vi "Write Stabilization Data.vi"(8 "error in (no error)":errorcluster, 9 "Output Path":path, 10 "Metadata Array":string[][](array[string]), 11 "Stabilization Data":T1={"Stabilization waveform"={"t0"=timestamp(0 s since 1904-01-01), "dt"=50.0, "Y"=[10.0, 9.0, 8.75, 8.5, 8.25, 8.125, 8.06, 8.03, 8.015, 8.0, 8.0, 8.0]}, "Variation"=0.0, "Stabilized"=FALSE, "Threshold"=0.0, "time to stabilize"=0.0, "3 points"=[], "Sphere Indicator"=enum."Naked Sphere"}) -> (0 "error out":errorcluster)   [LabVIEW 2014, in "Timing and Stabilization.lvlib"]
doc: "Save the details of the stabilization in a *.tdms file"
uses:
  Timing and Stabilization.lvlib
  Stabilization.ctl
  avantesSpectrometer/Acquisition/Sphere Indicator.ctl
  avantesSpectrometer/AvaSpec.lvlib
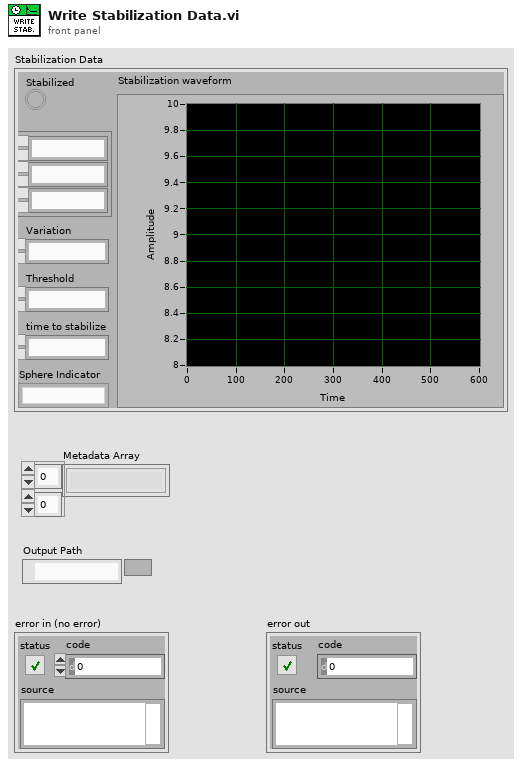
[diagram p1: front panel]
types:
  T1 = typedef "Timing and Stabilization.lvlib/Stabilization.ctl" = cluster{"Stabilization waveform":waveform(dbl), "Variation":dbl, "Stabilized":bool, "Threshold":dbl, "time to stabilize":dbl, "3 points":dbl[], "Sphere Indicator":T2}
  T2 = typedef "AvaSpec.lvlib/Sphere Indicator.ctl" = enum16{"Naked Sphere", "Insulated Sphere"}
  T3 = enum16{"open", "open or create", "create or replace", "create", "open (read-only)"}
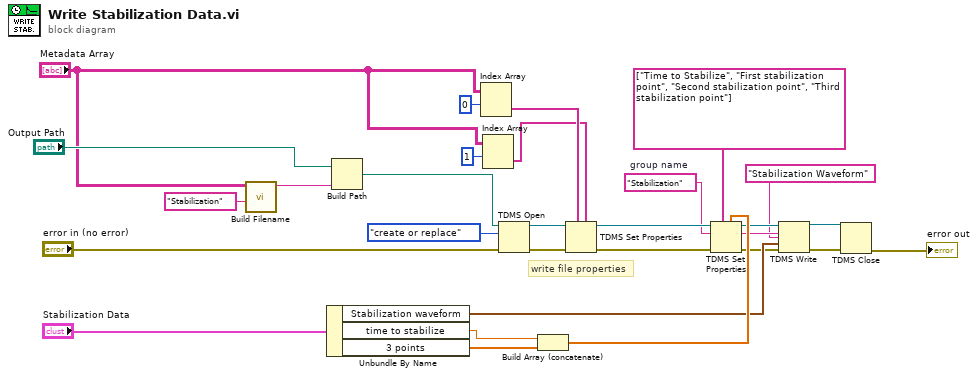
[diagram p0: block diagram]
diagram:
  w5 = "Stabilization"  # group name
  # "write file properties"
  n1 = call "Build Filename.vi"("Measurment Type"="Stabilization", "Metadata In"="Metadata Array") -> ("String"=w21:string)  [unwired: 9 in]
  n2 = Unbundle By Name("Stabilization Data") -> ("Stabilization waveform"=w25:waveform(dbl), "time to stabilize"=w28:dbl, "3 points"=w27:dbl[])
  n3 = Build Path(base path="Output Path", name or relative path=w21) -> (appended path=w9:path)
  n4 = Index Array(array="Metadata Array", index (row)=0) -> (element=w11:string[])  [unwired: 1 in]
  n5 = Index Array(array="Metadata Array", index (row)=1) -> (element=w10:string[])  [unwired: 1 in]
  n6 = TDMS Open(8:"error in (no error)", 10:T3."create or replace" ("operation (0:open)"), 11:w9) -> (0:w20:errorcluster, 3:w18:refnum<k34>)  [unwired: 4 in]
  n7 = Build Array (concatenate)(w28, w27) -> (w26:dbl[])
  n8 = TDMS Set Properties(5:w10, 7:w11, 8:w20, 11:w18) -> (0:w14:errorcluster, 3:w15:refnum<k34>)  [unwired: 2 in, 2 out]
  n9 = TDMS Set Properties(5:w26, 7:string[] ["Time to Stabilize", "First stabilization point", "Second stabilization point", "Third stabilization point"] ("property names"), 8:w14, 10:w5, 11:w15) -> (0:w7:errorcluster, 2:w8:string, 3:w6:refnum<k34>)  [unwired: 1 in, 1 out]
  n10 = TDMS Write(0:w6, 5:w8, 7:"Stabilization Waveform" ("channel name(s) in (Untitled)"), 9:w25, 11:w7) -> (4:w17:refnum<k34>, 15:w16:errorcluster)  [unwired: 1 in, 2 out]
  n11 = TDMS Close(8:w16, 11:w17) -> (0:→"error out":errorcluster)  [unwired: 1 out]
